vi "ADCP_Get_Data_Packet_Instance.vi"(8 "error in (no error)":errorcluster, 9 "Frame Index":i32=-1, 10 "Frame name":string, 11 "ADCP in":refnum<class "ADCP.lvclass">) -> (0 "error out":errorcluster, 2 "Data Packet":T2, 3 "ADCP out":refnum<class "ADCP.lvclass">)   [LabVIEW 2017, in "ADCP.lvclass"]
uses:
  ADCP.lvclass
  ADCP_Data_Packet_Transmit_Mode.ctl
  ADCP.lvclass/ADCP.ctl
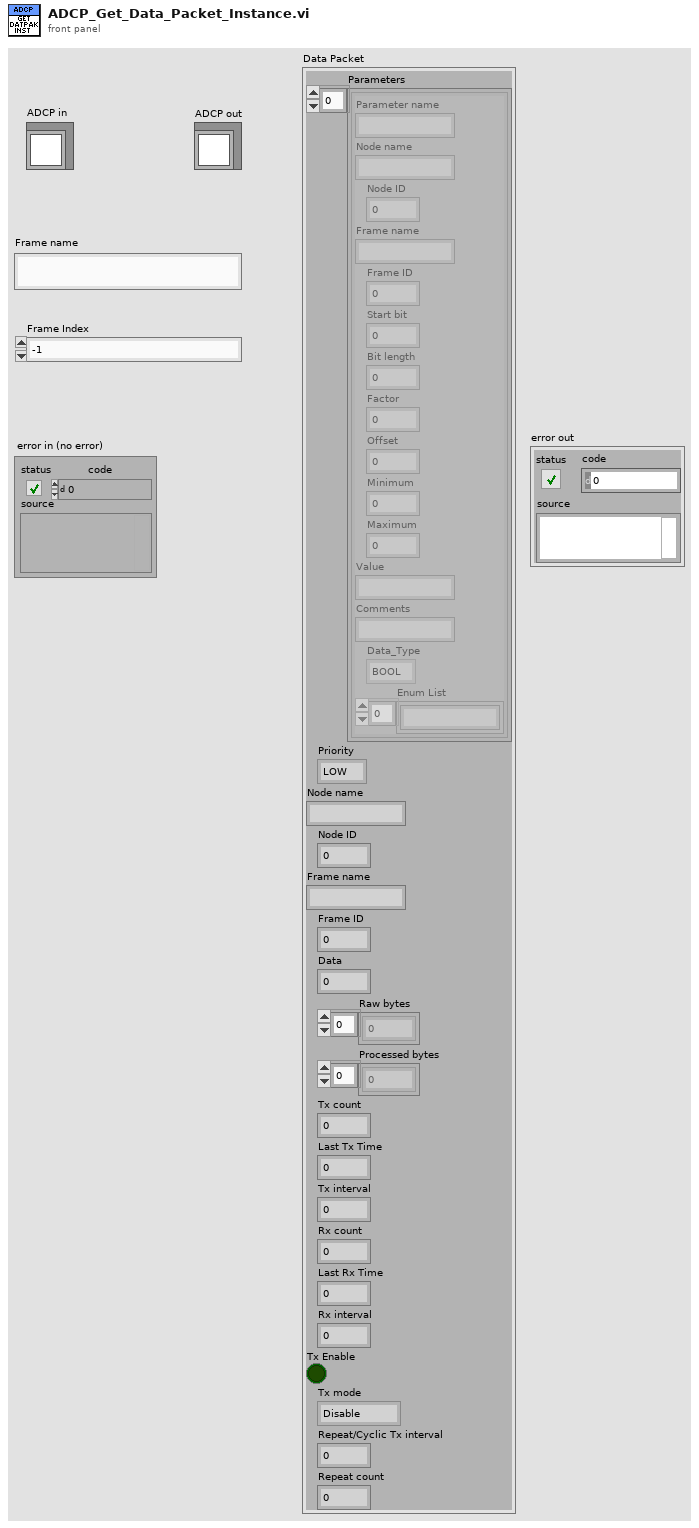
[diagram p1: front panel]
types:
  T1 = typedef "ADCP.lvclass/ADCP_Data_Packet_Transmit_Mode.ctl" = enum16{"Disable", "Single", "Cyclic", "Repeat"}
  T2 = cluster{"Parameters":cluster{"Parameter name":string, "Node name":string, "Node ID":u8, "Frame name":string, "Frame ID":u8, "Start bit":u32, "Bit length":u32, "Factor":dbl, "Offset":dbl, "Minimum":dbl, "Maximum":dbl, "Value":string, "Comments":string, "Data_Type":enum16{"BOOL", "UNSIGNED", "SIGNED", "FLOAT32", "ENUM"}, "Enum List":string[]}[], "Priority":enum16{"LOW", "HIGH"}, "Node name":string, "Node ID":u8, "Frame name":string, "Frame ID":u8, "Data":u32, "Raw bytes":u8[], "Processed bytes":u8[], "Tx count":i32, "Last Tx Time":u32, "Tx interval":u32, "Rx count":i32, "Last Rx Time":u32, "Rx interval":u32, "Tx Enable":bool, "Tx mode":T1, "Repeat/Cyclic Tx interval":u32, "Repeat count":u16}
  T3 = cluster{"Parameters":cluster{"Parameter name":string, "Node name":string, "Node ID":u8, "Frame name":string, "Frame ID":u8, "Start bit":u32, "Bit length":u32, "Factor":dbl, "Offset":dbl, "Minimum":dbl, "Maximum":dbl, "Value":string, "Comments":string, "Data_Type":enum16{"BOOL", "UNSIGNED", "SIGNED", "FLOAT32", "ENUM"}, "Enum List":string[]}[], "Priority":enum16{"LOW", "HIGH"}, "Node name":string, "Node ID":u8, "Frame name":string, "Frame ID":u8, "Data":u32, "Raw bytes":u8[], "Processed bytes":u8[], "Tx count":i32, "Last Tx Time":u32, "Tx interval":u32, "Rx count":i32, "Last Rx Time":u32, "Rx interval":u32, "Tx Enable":bool, "Tx mode":T1, "Repeat/Cyclic Tx interval":u32, "Repeat count":u16}[]
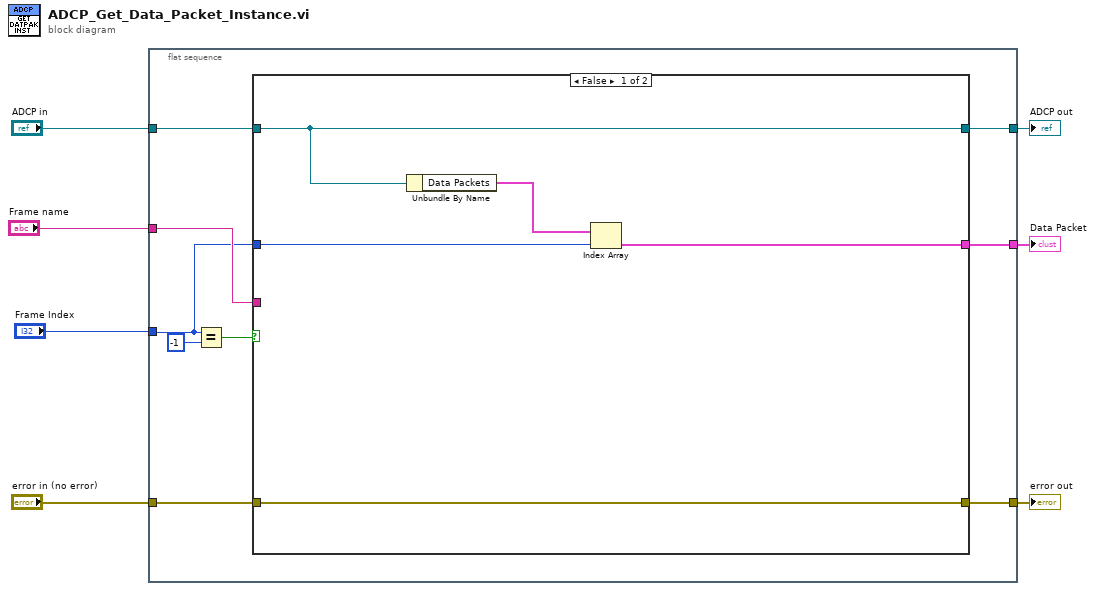
[diagram p0: block diagram]
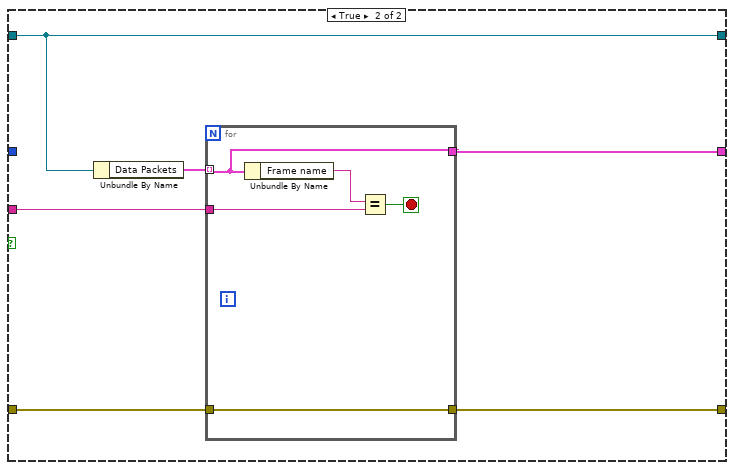
[diagram p2: hidden frame]
diagram:
  n1 = flat-sequence {
    tunnel: "ADCP in" -> [w14]
    tunnel: "Frame name" -> [w12]
    tunnel: "Frame Index" -> [w9]
    tunnel: "error in (no error)" -> [w13]
    tunnel: [w11] -> w2
    tunnel: [w10] -> w3
    tunnel: [w8] -> w1
    frame #0 {
      n2 = Equal?(x=w9, y=-1) -> (x = y?=w15:bool)
      n3 = case shown="False" w15 {
        tunnel: w14 -> [w17 w22]
        tunnel: w13 -> [w18 w27]
        tunnel: w12 -> [_ w25]
        tunnel: [w18 w24] -> w11
        tunnel: [w19 w23] -> w10
        tunnel: w9 -> [w20 _]
        tunnel: [w17 w22] -> w8
        frame False {
          n4 = Unbundle By Name(w17) -> ("Data Packets"=w21:T3)
          n5 = Index Array(array=w21, index=w20) -> (element=w19:T2)
        }
        frame True {
          n6 = Unbundle By Name(w22) -> ("Data Packets"=w26:T3)
          n7 = for {
            tunnel: w27 -> [w30]
            tunnel: w26 -> [w28] mode=indexing
            tunnel: w25 -> [w31]
            tunnel: [w30] -> w24
            tunnel: [w28] -> w23
            stop <- w29 stop-if-true
            n8 = Unbundle By Name(w28) -> ("Frame name"=w32:string)
            n9 = Equal?(x=w32, y=w31) -> (x = y?=w29:bool)
          }
        }
      }
    }
  }
  "Data Packet" <- w3
  "error out" <- w2
  "ADCP out" <- w1
